vi "Test 5.vi"(8 "error in (no error)":errorcluster, 11 "Test Case In":refnum<class "Tests.lvclass">) -> (0 "error out":errorcluster, 3 "Test Case Out":refnum<class "Tests.lvclass">)   [LabVIEW 2020, in "Tests.lvclass"]
uses:
  Tests.lvclass
  C:/Program Files (x86)/National Instruments/LabVIEW 2020/vi.lib/Astemes/LUnit/Test Case.lvclass
  <vilib>/Astemes/LUnit/Test Case.lvclass/Test Case.ctl
  4993e8ee-a06a-463a-9684-69129f64d5ce.vi
  <vilib>/Astemes/LUnit/Append Pass Result.vi
  <vilib>/Astemes/LUnit/Append Fail Result.vi
  <vilib>/Astemes/LUnit/Describe Comparison.vi
  <vilib>/Astemes/LUnit/Compare Variants.vi
  <vilib>/Astemes/LUnit/Variant to string.vi
  <vilib>/Utility/Data Type/Get Type Information.vi
  <vilib>/Utility/LVClass/Get LV Class Name.vi
  Proto/Group.lvclass
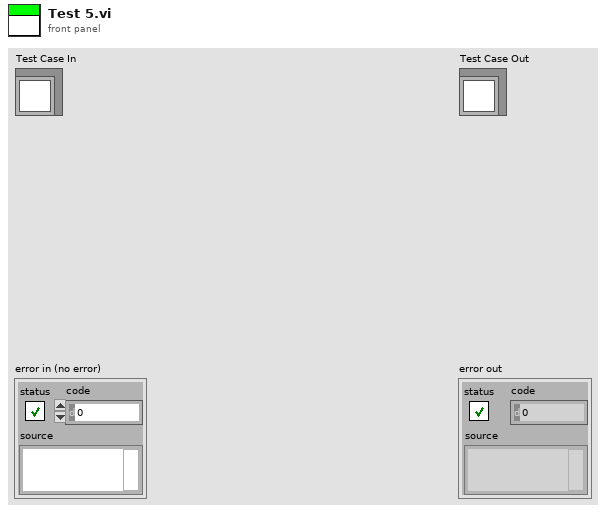
[diagram p1: front panel]
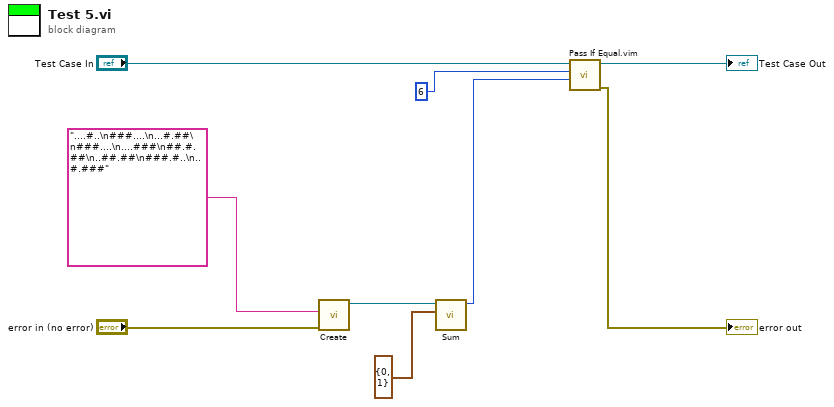
[diagram p0: block diagram]
diagram:
  n1 = call "Create.vi"("error in (no error)"="error in (no error)", "Input"="....#..\n###....\n...#.##\n###....\n....###\n##.#.##\n..##.##\n###.#..\n..#.###") -> ("Proto"=w2:refnum<class "Group.lvclass">)  [unwired: 8 in, 1 out]
  n2 = call "Sum.vi"("Reflections to ignore"=cluster{"Numeric":u64, "Numeric":u64} {"Numeric"=0, "Numeric"=1}, "Proto In"=w2) -> ("Numeric"=w4:u64)  [unwired: 8 in, 1 out]
  n3 = call "Pass If Equal.vim"("Actual"=w4, "Expected"=u64 6 ("Numeric"), "LUnit Test Case In"="Test Case In") -> ("error out"=→"error out":errorcluster, "LUnit Test Case Out"=→"Test Case Out":refnum<class "Tests.lvclass">)  [unwired: 7 in]
